vi "Periodic Tasks.vi"() -> ()   [LabVIEW 2011]
doc: "This VI runs in parallel to other tasks. It can contain as many user-defined periodic loops as you need. These can carry out PID or other sorts of timed response."
uses:
  <vilib>/Rock Robotics/SystemInterfaces/Utilities/FPGA_UtilitiesLED State.ctl
  <vilib>/Rock Robotics/SystemInterfaces/Utilities/FPGA_UtilitiesLED Source.ctl
  <vilib>/Platform/TimedLoop/XDataNode/timing_clust.ctl
  <vilib>/Platform/TimedLoop/XDataNode/nitl_modes.ctl
  <vilib>/Platform/TimedLoop/XDataNode/wakeup.ctl
  Robot Global Data.vi
  <vilib>/Platform/TimedLoop/XDataNode/XDataNode.xnode
  <vilib>/Platform/TimedLoop/XDataNode/XDNodeRunTimeDep.lvlib
panel:
  in  "error in (no error)":errorcluster
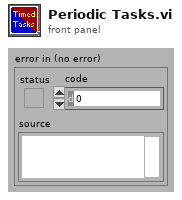
[diagram p1: front panel]
types:
  T1 = typedef "WPI_DriverStationRobotMode.ctl" = enum16{"Autonomous Disabled", "Autonomous Enabled", "Teleop Disabled", "Teleop Enabled", "Timeout", "Finish"}
  T2 = typedef "XDNodeRunTimeDep.lvlib/timing_clust.ctl" = cluster{"Expected End [f-1]":u64, "Actual End [f-1]":u64, "Finished Late? [f-1]":bool, "Expected End [i-1]":u64, "Actual End [i-1]":u64, "Finished Late? [i-1]":bool, "Expected Start [i]":u64, "Actual Start [i]":u64, "Expected Start [f]":u64, "Actual Start [f]":u64, "Source Name":string, "Structure Name":string, "Period":i64, "Deadline":i64, "Offset":i64, "Start":i64, "Priority":i32, "Timeout":i32, "Mode":T3, "Wakeup Reason":T4, "Error":errorcluster, "Source Type":string, "Secondary Source Type":string, "Global End Time":u64, "Global Start Time":u64, "Frame Duration":u64, "Iteration Duration":u64, "Assigned CPU":i32, "I/O Scan Engine Mode":u32}
  T3 = typedef "XDNodeRunTimeDep.lvlib/nitl_modes.ctl" = enum32{"No Change", "Process missed periods, maintain original phase", "Discard missed periods, maintain original phase", "Process missed periods, ignore original phase", "Discard missed periods, ignore original phase"}
  T4 = typedef "XDNodeRunTimeDep.lvlib/wakeup.ctl" = enum32{"Normal", "Aborted", "Asynchronous wakeup", "Timing source error", "Timed loop error", "Timeout"}
  T5 = typedef "FPGA_UtilitiesLED State.ctl" = enum16{"Off", "On", "Toggle"}
  T6 = typedef "FPGA_UtilitiesLED Source.ctl" = enum16{"User LED", "FPGA LED"}
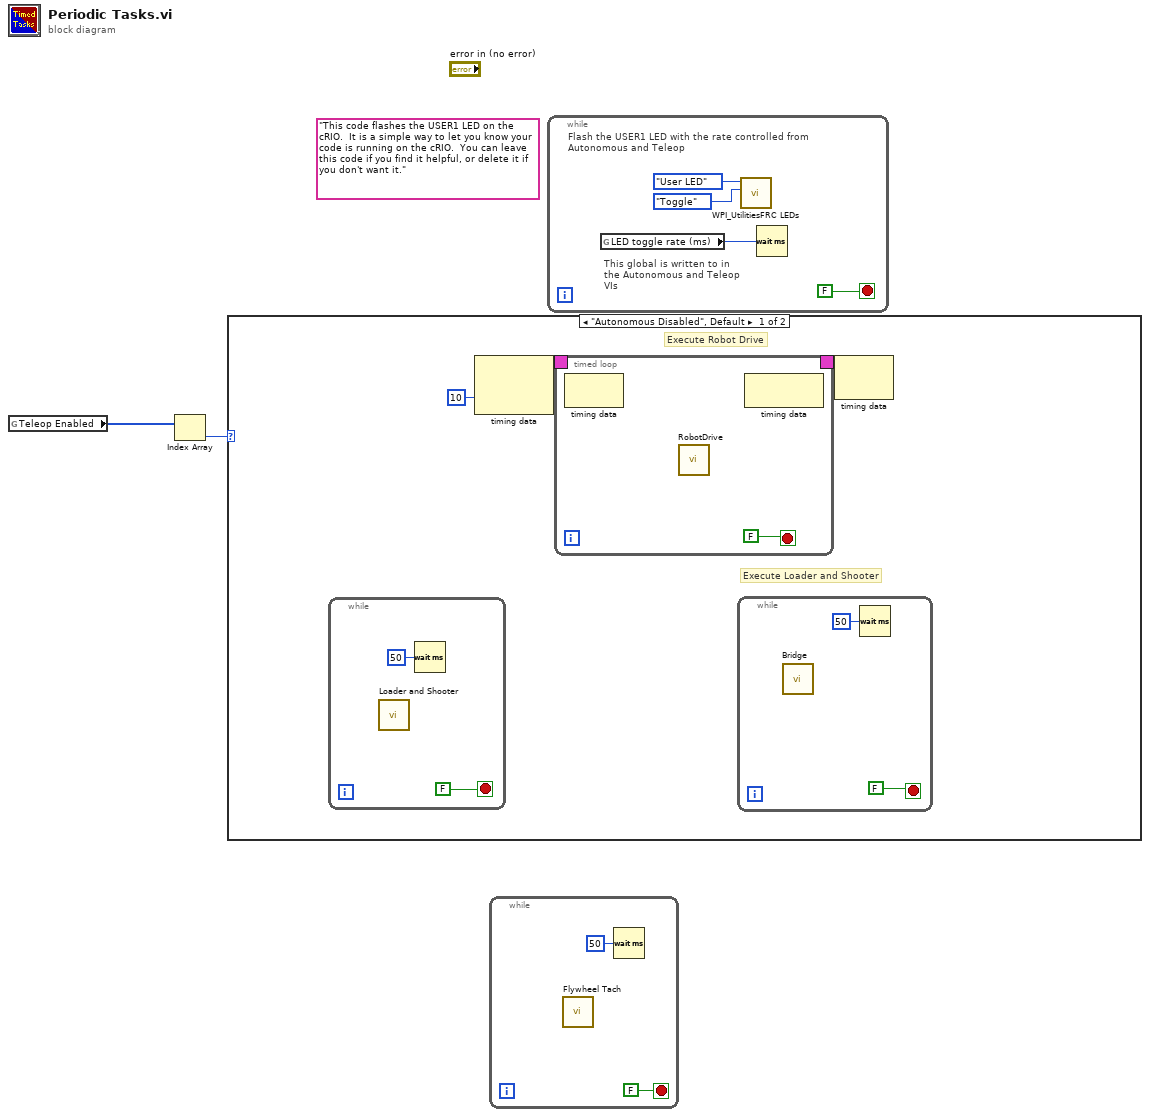
[diagram p0: block diagram]
diagram:
  (unwired) "This code flashes the USER1 LED on the cRIO.  It is a simple way to let you know your code is running on the cRIO.  You can leave this code if you find it helpful, or delete it if you don't want it."
  n1 = global read "Robot Global Data.vi" "Teleop Enabled"() -> (w2:T1[])
  n2 = Index Array "Index Array"(array=w2) -> (element=w1:T1)  [unwired: 1 in]
  n3 = case shown="\"Autonomous Disabled\", Default" w1 {
    frame "Autonomous Disabled", Default {
      # "Execute Loader and Shooter"
      # "Execute Robot Drive"
      n4 = while {
        stop <- FALSE stop-if-true
        n5 = call "Loader and Shooter.vi"() -> ()  [unwired: 12 in]
        n6 = Wait (ms)(milliseconds to wait=u32 50) -> ()  [unwired: 1 out]
      }
      n7 = node-c288(i64 10 ("Period")) -> (w5:T2)  [unwired: 1 in]
      n8 = timed-loop {
        timing: w5 -> [_]
        timing-out: [_] -> w4
        stop <- FALSE stop-if-true
        n9 = node-c288() -> ()  [unwired: 1 in, 1 out]
        n10 = call "RobotDrive.vi"() -> ()  [unwired: 12 in]
        n11 = node-c288() -> ()  [unwired: 1 in, 1 out]
      }
      n12 = while {
        stop <- FALSE stop-if-true
        n13 = call "Bridge.vi"() -> ()  [unwired: 12 in]
        n14 = Wait (ms)(milliseconds to wait=u32 50) -> ()  [unwired: 1 out]
      }
      n15 = node-c288(w4) -> ()  [unwired: 1 out]
    }
    frame "Autonomous Enabled" {
    }
  }
  n16 = while {
    stop <- FALSE stop-if-true
    n17 = call "Flywheel Tach.vi"() -> ()  [unwired: 12 in]
    n18 = Wait (ms)(milliseconds to wait=u32 50) -> ()  [unwired: 1 out]
  }
  n19 = while {
    stop <- FALSE stop-if-true
    # "This global is written to in the Autonomous and Teleop VIs"
    # "Flash the USER1 LED with the rate controlled from Autonomous and Teleop"
    n20 = global read "Robot Global Data.vi" "LED toggle rate (ms)"() -> (w19:u32)
    n21 = call <vilib>:"WPI_UtilitiesFRC LEDs.vi"("State"=FPGA_UtilitiesLED_State."Toggle", "LED Type"=FPGA_UtilitiesLED_Source."User LED") -> ()  [unwired: 1 in, 9 out]
    n22 = Wait (ms)(milliseconds to wait=w19) -> ()  [unwired: 1 out]
  }
